vi "SetTimer FGV.vi"(1 "Logging Rate":T1, 2 "sample interval (ms)":i32=50) -> (0 "Add?":bool=TRUE)   [LabVIEW 2018]
uses:
  Ctls/LoggingRate.ctl
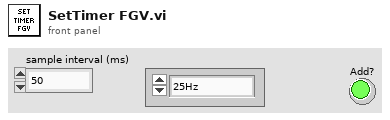
[diagram p1: front panel]
types:
  T1 = typedef "LoggingRate.ctl" = enum16{"25Hz", "30Hz", "35Hz", "40Hz"}
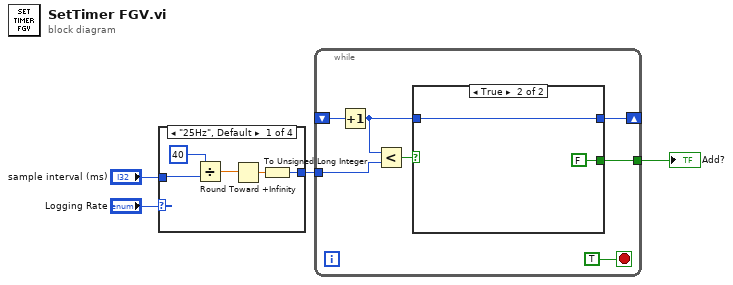
[diagram p0: block diagram]
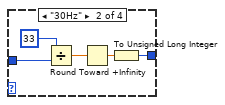
[diagram p2: hidden frame]
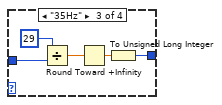
[diagram p3: hidden frame]
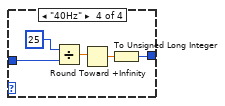
[diagram p4: hidden frame]
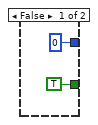
[diagram p5: hidden frame]
diagram:
  n1 = case shown="\"25Hz\", Default" "Logging Rate" {
    tunnel: "sample interval (ms)" -> [w8 w13 w18 w23]
    tunnel: [w5 w10 w15 w20] -> w1
    frame "25Hz", Default {
      n2 = Divide(x=40, y=w8) -> (x/y=w7:dbl)
      n3 = Round Toward +Infinity(x=w7) -> (ceil(x): smallest int >= x=w6:dbl)
      n4 = To Unsigned Long Integer(number=w6) -> (unsigned 32bit integer=w5:u32)
    }
    frame "30Hz" {
      n5 = Divide(x=33, y=w13) -> (x/y=w11:dbl)
      n6 = Round Toward +Infinity(x=w11) -> (ceil(x): smallest int >= x=w12:dbl)
      n7 = To Unsigned Long Integer(number=w12) -> (unsigned 32bit integer=w10:u32)
    }
    frame "35Hz" {
      n8 = Divide(x=29, y=w18) -> (x/y=w16:dbl)
      n9 = Round Toward +Infinity(x=w16) -> (ceil(x): smallest int >= x=w17:dbl)
      n10 = To Unsigned Long Integer(number=w17) -> (unsigned 32bit integer=w15:u32)
    }
    frame "40Hz" {
      n11 = Divide(x=25, y=w23) -> (x/y=w21:dbl)
      n12 = Round Toward +Infinity(x=w21) -> (ceil(x): smallest int >= x=w22:dbl)
      n13 = To Unsigned Long Integer(number=w22) -> (unsigned 32bit integer=w20:u32)
    }
  }
  n14 = while {
    shift-right: [w29] -> _
    shift-left: _ -> [w27]
    tunnel: [w28] -> w4
    tunnel: w1 -> [w25]
    stop <- TRUE stop-if-true
    n15 = Increment(x=w27) -> (x+1=w26:u32)
    n16 = Less?(x=w26, y=w25) -> (x < y?=w30:bool)
    n17 = case shown="True" w30 {
      tunnel: w26 -> [_ w34]
      tunnel: [u32 0 w34] -> w29
      tunnel: [TRUE FALSE] -> w28
      frame False {
      }
      frame True {
      }
    }
  }
  "Add?" <- w4
